vi "Search Sorted Table 1st Col.vi"(10 "Seach Value":string, 11 "Table to Search":string[][](array[string])) -> (3 "Search Result":string[][](array[string]))   [LabVIEW 2009]
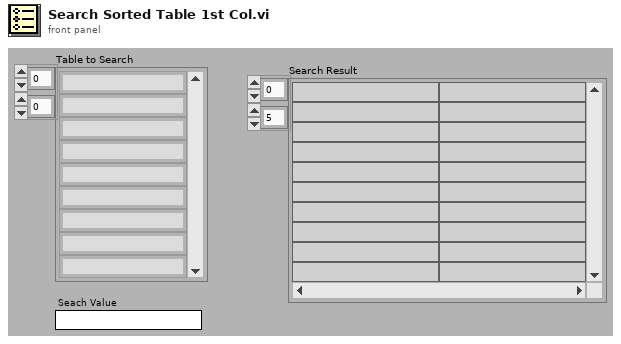
[diagram p1: front panel]
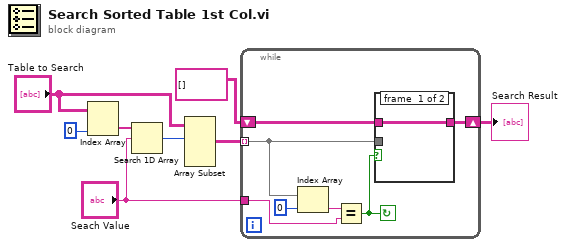
[diagram p0: block diagram]
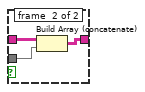
[diagram p2: hidden frame]
diagram:
  n1 = Index Array(array="Table to Search", index (col)=0 ("disabled index (col)")) -> (element=w7:string[])  [unwired: 1 in]
  n2 = Search 1D Array(1D array=w7, element="Seach Value") -> (index of element=w5:i32)  [unwired: 1 in]
  n3 = Array Subset(array="Table to Search", index (row)=w5) -> (w4:string[][])  [unwired: 3 in]
  n4 = while {
    tunnel: w4 -> [w12] mode=indexing
    tunnel: "Seach Value" -> [w13]
    shift-right: [w11] -> w1
    shift-left: string[][] [] -> [w10]
    stop <- w9 continue-if-true
    n5 = Index Array(array=w12, index=0) -> (element=w14:string)
    n6 = Equal?(x=w14, y=w13) -> (x = y?=w9:bool)
    n7 = case shown="True" w9 {
      tunnel: w12 -> [_ w19]
      tunnel: [w16 w18] -> w11
      tunnel: w10 -> [w16 w17]
      frame #0 {
      }
      frame #1 {
        n8 = Build Array (concatenate)(w17, w19) -> (w18:string[][])
      }
    }
  }
  "Search Result" <- w1
